vi "User Add.vi"(8 "error in (no error)":errorcluster, 10 "User Record":T2, 11 "Connection Refnum":T1) -> (0 "error out":errorcluster, 2 "New User Record":T2, 3 "Connection Refnum":T1)   [LabVIEW 2011]
uses:
  User Record.ctl
  SI.LIB/ODBC/SQL Controls/Connection Refnum.ctl
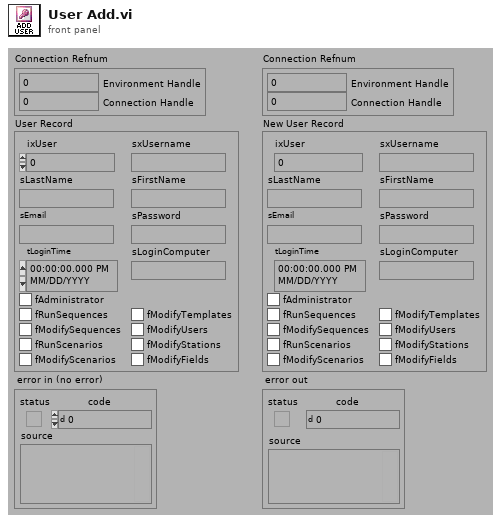
[diagram p1: front panel]
types:
  T1 = typedef "Connection Refnum.ctl" = cluster{"Environment Handle":i32, "Connection Handle":i32}
  T2 = typedef "User Record.ctl" = cluster{"ixUser":i32, "sxUsername":string, "sLastName":string, "sFirstName":string, "sEmail":string, "sPassword":string, "tLoginTime":timestamp, "sLoginComputer":string, "fAdministrator":bool, "fRunSequences":bool, "fModifySequences":bool, "fRunScenarios":bool, "fModifyScenarios":bool, "fModifyTemplates":bool, "fModifyUsers":bool, "fModifyStations":bool, "fModifyFields":bool}
  T3 = typedef "Statement Refnum.ctl" = cluster{"Statement Handle":i32, "Parameter Number":u16}
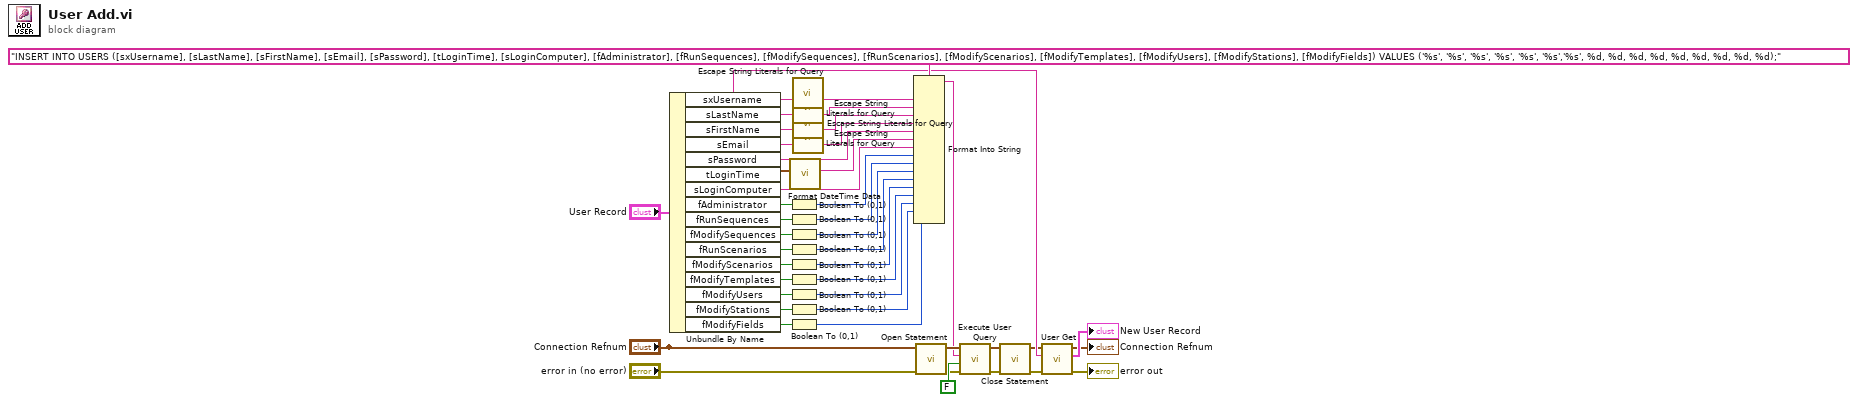
[diagram p0: block diagram]
diagram:
  n1 = Unbundle By Name("User Record") -> ("sxUsername"=w3:string, "sLastName"=w31:string, "sFirstName"=w30:string, "sEmail"=w29:string, "sPassword"=w14:string, "tLoginTime"=w25:timestamp, "sLoginComputer"=w28:string, "fAdministrator"=w15:bool, "fRunSequences"=w16:bool, "fModifySequences"=w17:bool, "fRunScenarios"=w18:bool, "fModifyScenarios"=w19:bool, "fModifyTemplates"=w20:bool, "fModifyUsers"=w21:bool, "fModifyStations"=w22:bool, "fModifyFields"=w23:bool)
  n2 = Boolean To (0,1)(Boolean=w15) -> (0, 1=w13:i16)
  n3 = Boolean To (0,1)(Boolean=w16) -> (0, 1=w12:i16)
  n4 = Boolean To (0,1)(Boolean=w17) -> (0, 1=w11:i16)
  n5 = Boolean To (0,1)(Boolean=w18) -> (0, 1=w10:i16)
  n6 = Boolean To (0,1)(Boolean=w19) -> (0, 1=w9:i16)
  n7 = Boolean To (0,1)(Boolean=w20) -> (0, 1=w8:i16)
  n8 = Boolean To (0,1)(Boolean=w21) -> (0, 1=w7:i16)
  n9 = Boolean To (0,1)(Boolean=w22) -> (0, 1=w6:i16)
  n10 = Boolean To (0,1)(Boolean=w23) -> (0, 1=w5:i16)
  n11 = call "Format DateTime Data.vi"("Timestamp in"=w25) -> ("UTC DB String out"=w24:string)  [unwired: 10 out]
  n12 = call "Escape String Literals for Query.vi"("String"=w3) -> ("escaped String"=w35:string)  [unwired: 1 in, 13 out]
  n13 = call "Escape String Literals for Query.vi"("String"=w31) -> ("escaped String"=w34:string)  [unwired: 1 in, 13 out]
  n14 = call "Escape String Literals for Query.vi"("String"=w30) -> ("escaped String"=w33:string)  [unwired: 1 in, 13 out]
  n15 = call "Escape String Literals for Query.vi"("String"=w29) -> ("escaped String"=w32:string)  [unwired: 1 in, 13 out]
  n16 = Format Into String(format string="INSERT INTO USERS ([sxUsername], [sLastName], [sFirstName], [sEmail], [sPassword], [tLoginTime], [sLoginComputer], [fAdministrator], [fRunSequences], [fModifySequences], [fRunScenarios], [fModifyScenarios], [fModifyTemplates], [fModifyUsers], [fModifyStations], [fModifyFields]) VALUES ('%s', '%s', '%s', '%s', '%s', '%s','%s', %d, %d, %d, %d, %d, %d, %d, %d, %d);" ("User Query"), w35, w34, w33, w32, w14, w24, w28, w13, w12, w11, w10, w9, w8, w7, w6, w5) -> (resulting string=w37:string)  [unwired: 2 in, 1 out]
  n17 = call "Open Statement.vi"("error in (no error)"="error in (no error)", "Connection Refnum"="Connection Refnum") -> ("error out"=w39:errorcluster, "Statement Refnum"=w38:T3)  [unwired: 4 out]
  n18 = call "Execute User Query.vi"("error in (no error)"=w39, "Return Data? (f)"=FALSE, "User Query"=w37, "Statement Refnum"=w38) -> ("error out"=w41:errorcluster, "Statement Refnum"=w42:T3)  [unwired: 2 out]
  n19 = call "Close Statement.vi"("error in (no error)"=w41, "Statement Refnum"=w42) -> ("error out"=w36:errorcluster)  [unwired: 5 out]
  n20 = call "User Get.vi"("error in (no error)"=w36, "sxUsername (\"\")"=w3, "Connection Refnum"="Connection Refnum") -> ("error out"=→"error out":errorcluster, "User"=→"New User Record":T2, "Connection Refnum"=→"Connection Refnum":T1)  [unwired: 6 out]
